vi "StepperMotorDriver.vi"(6 "pCoordinate":refnum<vi>, 8 "error in":errorcluster, 9 "Dinstance Multiplier":i32=40, 10 "Distance":dbl, 11 "Direction":u16(ring) items=["x", "y"]) -> (0 "error out":errorcluster)   [LabVIEW 2021]
uses:
  <vilib>/DAQmx/write.llb/DAQmx Write (Digital Bool 1Line 1Point).vi
  <vilib>/DAQmx/create/channels.llb/DAQmx Create Channel (DO-Digital Output).vi
  <vilib>/DAQmx/miscellaneous.llb/DAQmx Fill In Error Info.vi
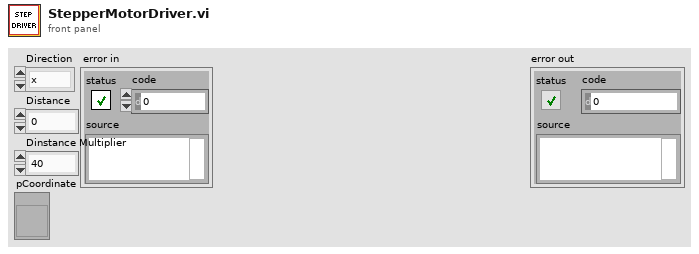
[diagram p1: front panel]
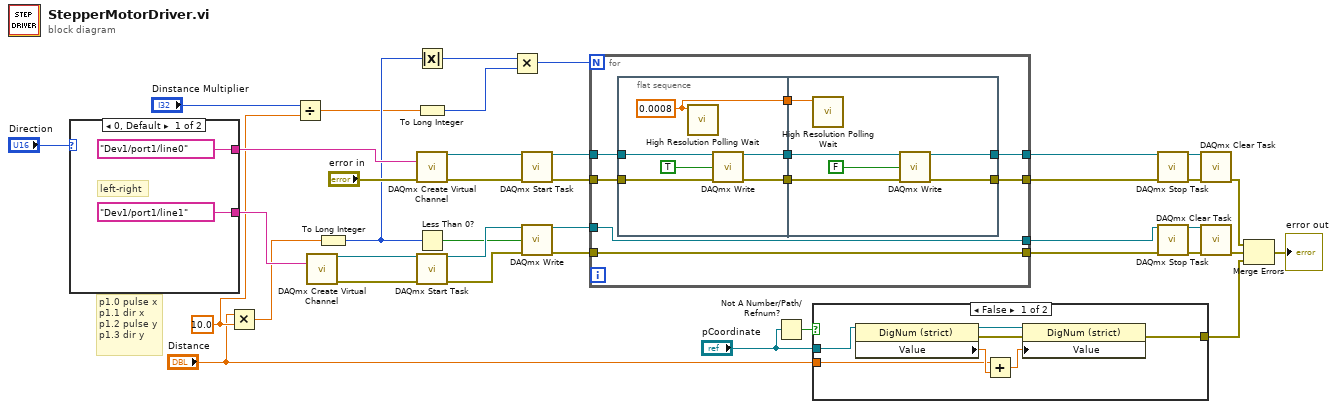
[diagram p0: block diagram]
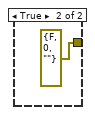
[diagram p2: hidden frame]
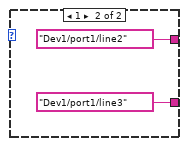
[diagram p3: hidden frame]
diagram:
  w7 = 10.0 ("y")
  # "p1.0 pulse x\np1.1 dir x\np1.2 pulse y\np1.3 dir y"
  n1 = case shown="0, Default" "Direction" {
    tunnel: [tag "Dev1/port1/line0" ("lines") tag "Dev1/port1/line2" ("lines")] -> w17
    tunnel: [tag "Dev1/port1/line1" ("lines") tag "Dev1/port1/line3" ("lines")] -> w16
    frame 0, Default {
      # "left-right"
    }
    frame 1 {
    }
  }
  n2 = Multiply(x="Distance", y=w7) -> (x*y=w10:dbl)
  n3 = Divide(x="Dinstance Multiplier", y=w7) -> (x/y=w6:dbl)
  n4 = call-poly <vilib>:"DAQmx Create Virtual Channel.vi"("lines"=w16) -> ("task out"=w34:refnum<k21>, "error out"=w33:errorcluster)  [unwired: 13 in]
  n5 = To Long Integer(number=w10) -> (32bit integer=w9:i32)
  n6 = Absolute Value(x=w9) -> (abs(x)=w11:i32)
  n7 = To Long Integer(number=w6) -> (32bit integer=w5:i32)
  n8 = call-poly <vilib>:"DAQmx Create Virtual Channel.vi"("lines"=w17, "error in"="error in") -> ("task out"=w36:refnum<k21>, "error out"=w35:errorcluster)  [unwired: 12 in]
  n9 = Less Than 0?(x=w9) -> (x < 0?=w12:bool)
  n10 = call <vilib>:"DAQmx Start Task.vi"("task/channels in"=w34, "error in"=w33) -> ("task out"=w32:refnum<k21>, "error out"=w31:errorcluster)  [unwired: 12 in]
  n11 = Multiply(x=w11, y=w5) -> (x*y=w15:i32)
  n12 = call <vilib>:"DAQmx Start Task.vi"("task/channels in"=w36, "error in"=w35) -> ("task out"=w38:refnum<k21>, "error out"=w37:errorcluster)  [unwired: 12 in]
  n13 = call-poly <vilib>:"DAQmx Write.vi"("task/channels in"=w32, "data"=w12, "error in"=w31) -> ("task out"=w26:refnum<k21>, "error out"=w25:errorcluster)  [unwired: 10 in, 1 out]
  n14 = for {
    N: w15 -> [_]
    tunnel: w25 -> [w44]
    tunnel: [w44] -> w27
    tunnel: w26 -> [w45]
    tunnel: [w45] -> w28
    tunnel: w37 -> [w48]
    tunnel: [w46] -> w29
    tunnel: w38 -> [w49]
    tunnel: [w47] -> w30
    n15 = flat-sequence {
      tunnel: w49 -> [w57]
      tunnel: w48 -> [w56]
      tunnel: [w55] -> w51
      tunnel: [w54] -> w50
      tunnel: [w52] -> w43
      tunnel: w51 -> [w63]
      tunnel: w50 -> [w62]
      tunnel: [w61] -> w47
      tunnel: [w60] -> w46
      tunnel: w43 -> [w58]
      frame #0 {
        w52 = 0.0008 ("seconds to wait")
        n16 = call <vilib>:"High Resolution Polling Wait.vi"("seconds to wait"=w52) -> ()  [unwired: 10 in, 1 out]
        n17 = call-poly <vilib>:"DAQmx Write.vi"("task/channels in"=w57, "data"=TRUE, "error in"=w56) -> ("task out"=w55:refnum<k21>, "error out"=w54:errorcluster)  [unwired: 10 in, 1 out]
      }
      frame #1 {
        n18 = call <vilib>:"High Resolution Polling Wait.vi"("seconds to wait"=w58) -> ()  [unwired: 10 in, 1 out]
        n19 = call-poly <vilib>:"DAQmx Write.vi"("task/channels in"=w63, "data"=FALSE, "error in"=w62) -> ("task out"=w61:refnum<k21>, "error out"=w60:errorcluster)  [unwired: 10 in, 1 out]
      }
    }
  }
  n20 = Not A Number/Path/Refnum?(number/path/refnum="pCoordinate") -> (NaN/Path/Refnum?=w1:bool)
  n21 = case shown="False" w1 {
    tunnel: "Distance" -> [w66 _]
    tunnel: "pCoordinate" -> [w65 _]
    tunnel: [w64 errorcluster {"status"=FALSE, "code"=0, "source"=""} ("error out")] -> w2
    frame False {
      n22 = property class="DigNum (strict)"(reference=w65) -> (reference out=w67:refnum<vi>, error out=w70:errorcluster, "Value"=w68:dbl)  [unwired: 1 in]
      n23 = Add(x=w66, y=w68) -> (x+y=w69:dbl)
      n24 = property class="DigNum (strict)"(reference=w67, error in=w70, "Value"=w69) -> (error out=w64:errorcluster)  [unwired: 1 out]
    }
    frame True {
    }
  }
  n25 = call <vilib>:"DAQmx Stop Task.vi"("task/channels in"=w30, "error in"=w29) -> ("task out"=w24:refnum<k21>, "error out"=w23:errorcluster)  [unwired: 12 in]
  n26 = call <vilib>:"DAQmx Stop Task.vi"("task/channels in"=w28, "error in"=w27) -> ("task out"=w22:refnum<k21>, "error out"=w21:errorcluster)  [unwired: 12 in]
  n27 = call <vilib>:"DAQmx Clear Task.vi"("task in"=w24, "error in"=w23) -> ("error out"=w20:errorcluster)  [unwired: 13 in]
  n28 = call <vilib>:"DAQmx Clear Task.vi"("task in"=w22, "error in"=w21) -> ("error out"=w19:errorcluster)  [unwired: 13 in]
  n29 = Merge Errors(w20, w19, w2) -> (→"error out":errorcluster)
